vi "0+...+100.vi"() -> ()   [LabVIEW 2018]
panel:
  out "x+y":i32
  out "数值":i32
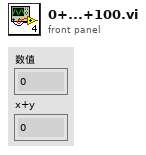
[diagram p1: front panel]
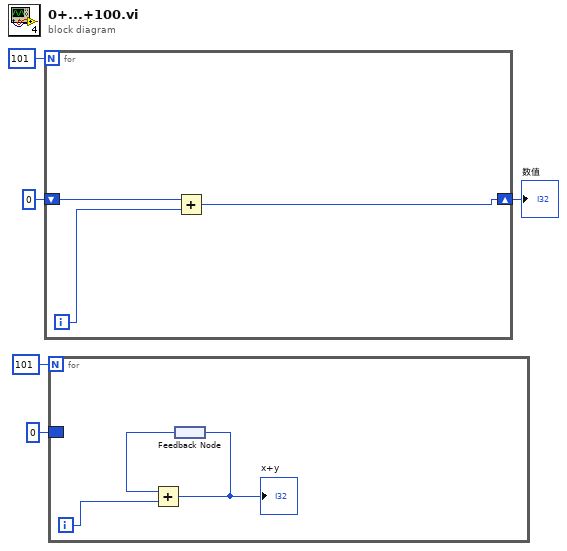
[diagram p0: block diagram]
diagram:
  n1 = for {
    N: 101 -> [_]
    shift-right: [w7] -> w3
    shift-left: 0 -> [w6]
    i -> [w8]
    n2 = Add(x=w6, y=w8) -> (x+y=w7:i32)
  }
  "数值" <- w3
  n3 = for {
    N: 101 -> [_]
    border: 0 -> [_]
    i -> [w11]
    n4 = feedback #1() -> (w9:i32)
    n5 = Add(x=w9, y=w11) -> (x+y=w10:i32)
    "x+y" <- w10
    n6 = feedback-in #1(w10) -> ()
  }
